vi "get_indices.vi"(8 "error in (no error)":errorcluster, 11 "Interface_get_indices in":refnum<class "Interface_get_indices.lvclass">) -> (0 "error out":errorcluster, 2 "out":cluster{"row_ind":dbl, "col_ind":dbl}, 3 "Interface_get_indices out":refnum<class "Interface_get_indices.lvclass">)   [LabVIEW 2020, in "Interface_get_indices.lvclass"]
doc: "Row and column indices of the i’th bicluster.\n\nOnly works if rows_ and columns_ attributes exist."
uses:
  Interface_get_indices.lvclass
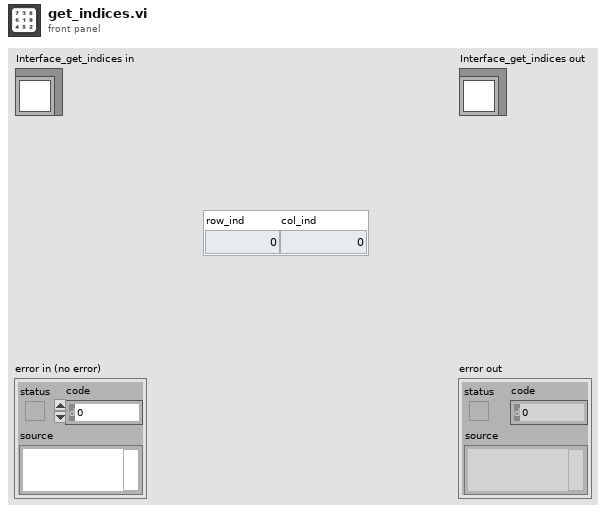
[diagram p1: front panel]
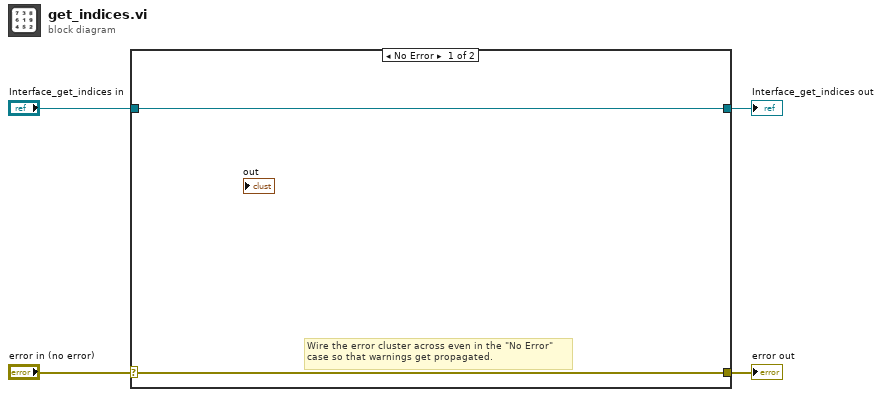
[diagram p0: block diagram]
diagram:
  n1 = case shown="No Error" "error in (no error)" {
    selector: "error in (no error)" -> [w5 w8]
    tunnel: [w5 w8] -> w3
    tunnel: [w6 w7] -> w1
    tunnel: "Interface_get_indices in" -> [w6 w7]
    frame No Error {
      # "Wire the error cluster across even in the \"No Error\"\ncase so that warnings get propagated."
    }
    frame Error {
    }
  }
  "error out" <- w3
  "Interface_get_indices out" <- w1
